vi "ConnectBySerialNumber.vi"(8 "error in":errorcluster, 11 "AdapterSerialNumber":string) -> (0 "error out":errorcluster, 3 "CanHandleOut":T1)   [LabVIEW 2011, in "Konvolucio MCAN120803.lvlib"]
doc: "Connect the adapter using the serial number."
uses:
  <instrlib>/Konvolucio MCAN120803/Konvolucio MCAN120803.lvlib
  <instrlib>/Konvolucio MCAN120803/Types/CanHandleType.ctl
  C:/Program Files/National Instruments/LabVIEW 2011/instr.lib/Konvolucio MCAN120803/Private/Konvolucio.MCAN120803.API.dll
  Private/Konvolucio.MCAN120803.API.dll
  <instrlib>/Konvolucio MCAN120803/Types/StateType.ctl
  <instrlib>/Konvolucio MCAN120803/Public/Attributes/AttrGetState.vi
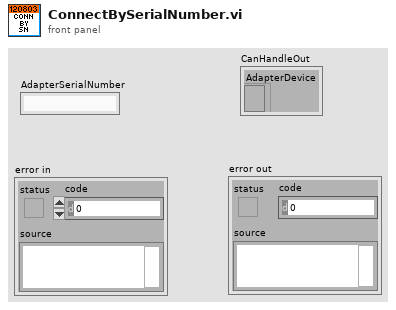
[diagram p1: front panel]
types:
  T1 = typedef "Konvolucio MCAN120803.lvlib/CanHandleType.ctl" = cluster{"AdapterDevice":refnum<k24>}
  T2 = typedef "Konvolucio MCAN120803.lvlib/StateType.ctl" = enum16{"SDEV_NONE", "SDEV_START", "SDEV_STOP", "SDEV_RESET", "SDEV_FAIL", "SDEV_IDLE"}
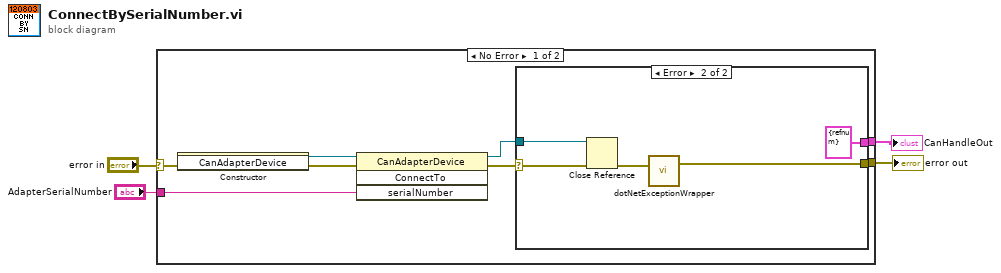
[diagram p0: block diagram]
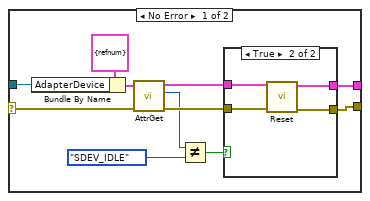
[diagram p2: hidden frame]
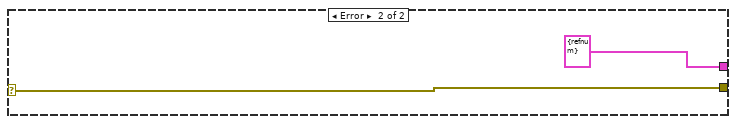
[diagram p4: hidden frame]
diagram:
  n1 = case shown="No Error" "error in" {
    selector: "error in" -> [w10 w36]
    tunnel: "AdapterSerialNumber" -> [w6 _]
    tunnel: [w5 T1 {"AdapterDevice"=refnum} ("HandleOut")] -> w2
    tunnel: [w7 w36] -> w1
    frame No Error {
      n2 = constructor class="CanAdapterDevice" ("MCanAdapter")(error in=w10) -> (reference out=w11:refnum<k24>, error out=w12:errorcluster)  [unwired: 2 in, 1 out]
      n3 = invoke class="CanAdapterDevice" method="ConnectTo"(reference=w11, error in=w12, "serialNumber"=w6) -> (reference out=w8:refnum<k24>, error out=w9:errorcluster)  [unwired: 1 in, 2 out]
      n4 = case shown="Error" w9 {
        selector: w9 -> [w15 w33]
        tunnel: w8 -> [w22 w34]
        tunnel: [w14 w31] -> w7
        tunnel: [w13 T1 {"AdapterDevice"=refnum} ("MCanHandleOut")] -> w5
        frame No Error {
          n5 = Bundle By Name(cluster=T1 {"AdapterDevice"=refnum}, "AdapterDevice"=w22) -> (w16:T1)
          n6 = call-poly <instrlib>:"AttrGet.vi"("error in"=w15, "CanHandleIn"=w16) -> ("error out"=w20:errorcluster, "State"=w18:T2, "CanHandleOut"=w21:T1)  [unwired: 7 in]
          n7 = Not Equal?(x=w18, y=StateType."SDEV_IDLE") -> (x != y?=w19:bool)
          n8 = case shown="True" w19 {
            tunnel: w20 -> [w24 w29]
            tunnel: w21 -> [w25 w28]
            tunnel: [w25 w27] -> w13
            tunnel: [w24 w26] -> w14
            frame False {
            }
            frame True {
              n9 = call <instrlib>:"Reset.vi"("error in"=w29, "CanHandleIn"=w28) -> ("error out"=w26:errorcluster, "CanHandleOut"=w27:T1)  [unwired: 8 in]
            }
          }
        }
        frame Error {
          n10 = Close Reference(reference=w34, error in (no error)=w33) -> (error out=w32:errorcluster)
          n11 = call <instrlib>:"dotNetExceptionWrapper.vi"("error in"=w32) -> ("error out"=w31:errorcluster)  [unwired: 2 in]
        }
      }
    }
    frame Error {
    }
  }
  "error out" <- w1
  "CanHandleOut" <- w2
